vi "FTW-VIServer-LabVIEWinfo.vi"(11 "error in":errorcluster) -> (4 "LabVIEW Version Year":string, 6 "LabVIEW Version Number":string, 8 "LabVIEW Display Version":string, 15 "error out":errorcluster)   [LabVIEW 2012]
panel:
  # "Inputs"
  # "Outputs"
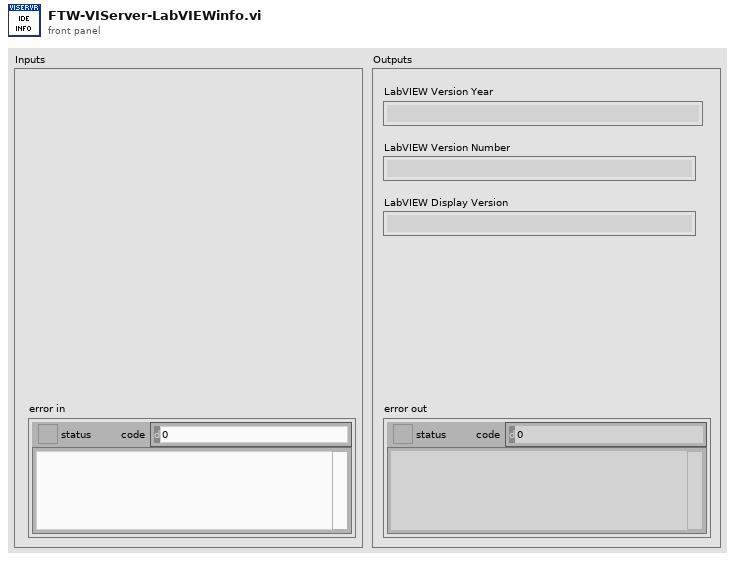
[diagram p1: front panel]
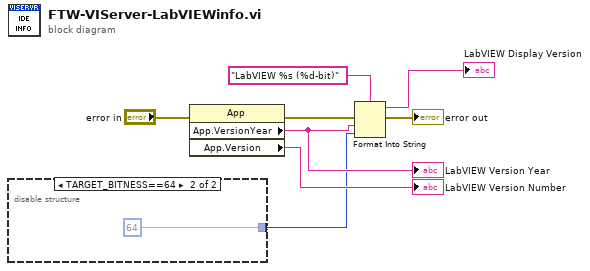
[diagram p0: block diagram]
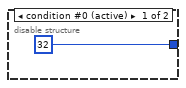
[diagram p2: hidden frame]
diagram:
  n1 = disable-structure shown="TARGET_BITNESS==64" {
    disable-tunnel: [32 ("input 2") 64 ("input 2")] -> w1
    frame condition #0 (active) {
    }
    frame condition #1 {
    }
  }
  n2 = property class="App"(error in="error in") -> (error out=w6:errorcluster, "App.VersionYear"=w3:string, "App.Version"=→"LabVIEW Version Number":string)  [unwired: 1 in, 1 out]
  "LabVIEW Version Year" <- w3
  n3 = Format Into String(format string="LabVIEW %s (%d-bit)", error in=w6, w3, w1) -> (resulting string=→"LabVIEW Display Version":string, error out=→"error out":errorcluster)  [unwired: 1 in]
